vi "_PC_Pub ctrlRegistry.vi"(5 "type":enum16{"None", "Write", "Read"}(ring)=enum."Read", 7 "function":T1=enum."ExeStatu", 8 "error in (no error)":errorcluster, 10 "node":string, 11 "write value":variant) -> (0 "error out":errorcluster, 1 "Boolean output":bool, 2 "SZ output":string, 3 "DWORD outpur":u32)   [LabVIEW 2018]
uses:
  Ctl/RegistyFunc.ctl
  <vilib>/registry/registry.llb/Registry RtKey.ctl
  <vilib>/registry/registry.llb/Read Registry Value Simple U32.vi
  <vilib>/registry/registry.llb/Write Registry Value Simple U32.vi
  <vilib>/registry/registry.llb/Read Registry Value Simple STR.vi
  <vilib>/registry/registry.llb/Write Registry Value Simple STR.vi
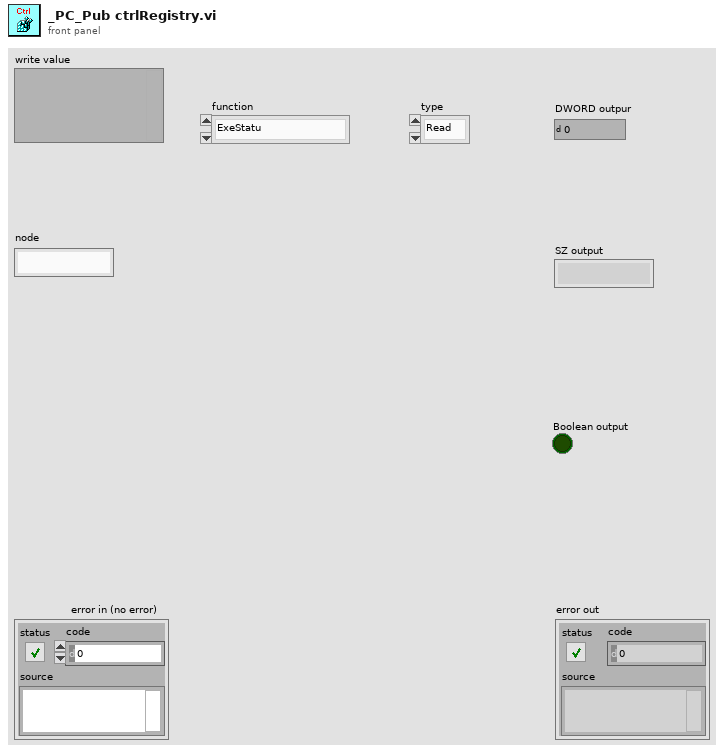
[diagram p1: front panel]
types:
  T1 = typedef "RegistyFunc.ctl" = enum16{"None", "FileAutoSave", "FileNoise", "FileSN", "ExeStatu", "WorkFolderPath", "MethodPath", "AVGItem", "LoopItem", "AutoRun", "BGColor", "LineColor", "LineWidth", "XGrid", "YGrid", "DeviceRefnum"}
  T2 = typedef "Registry RtKey.ctl" = enum32{"HKEY_CLASSES_ROOT", "HKEY_CURRENT_USER", "HKEY_LOCAL_MACHINE", "HKEY_USERS", "HKEY_PERFORMANCE_DATA", "HKEY_CURRENT_CONFIG", "HKEY_DYN_DATA"}
  T3 = typedef "Registry refnum.ctl" = refnum<k1>
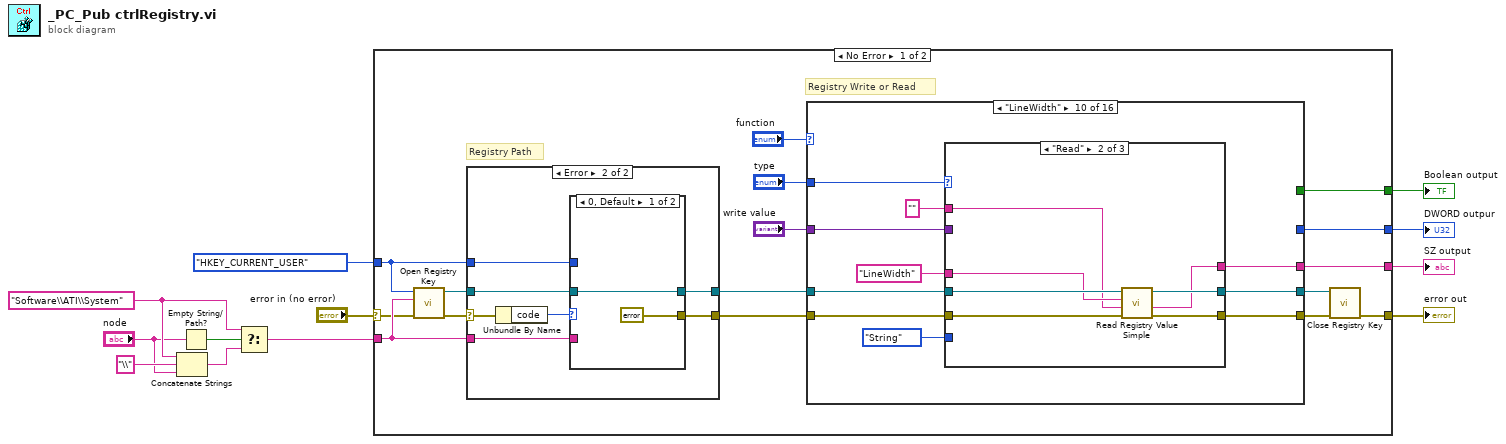
[diagram p0: block diagram]
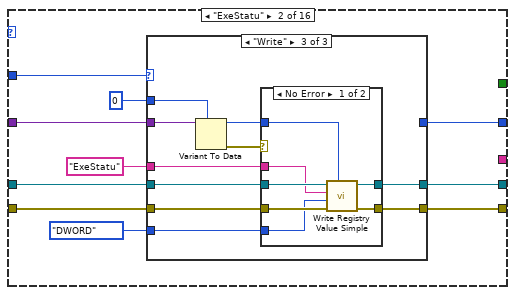
[diagram p3: hidden frame]
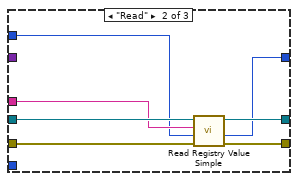
[diagram p5: hidden frame]
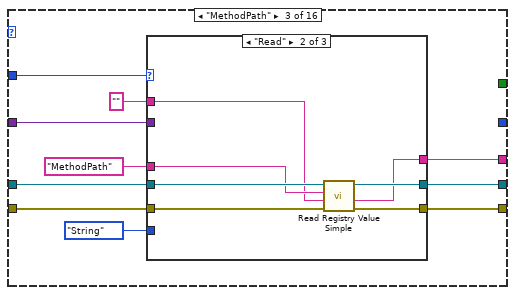
[diagram p7: hidden frame]
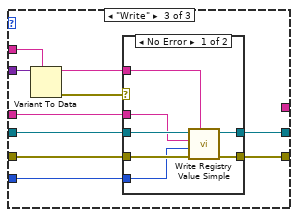
[diagram p9: hidden frame]
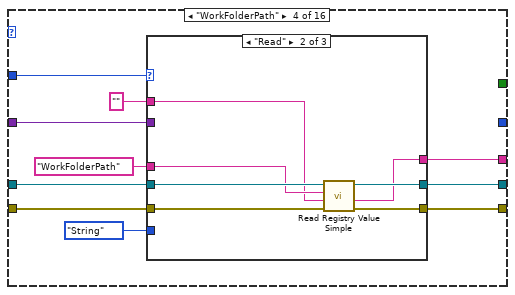
[diagram p11: hidden frame]
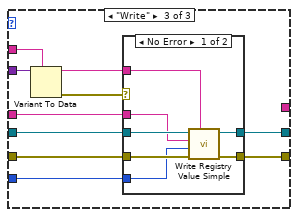
[diagram p13: hidden frame]
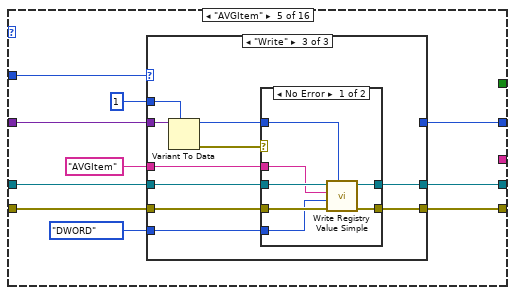
[diagram p15: hidden frame]
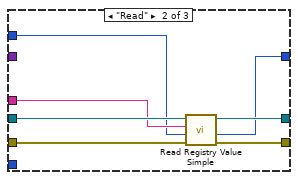
[diagram p17: hidden frame]
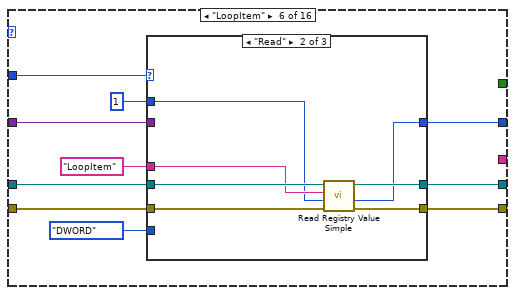
[diagram p19: hidden frame]
diagram:
  w9 = "Software\\ATI\\System" ("subkey")
  n1 = Concatenate Strings(w9, "\\" ("string"), "node") -> (w6:string)
  n2 = Empty String/Path?(string/path="node") -> (empty?=w10:bool)
  n3 = Select(t=w9, s=w10, f=w6) -> (s? t:f=w5:string)
  n4 = case shown="No Error" "error in (no error)" {
    selector: "error in (no error)" -> [w13 w636]
    tunnel: Registry_RtKey."HKEY_CURRENT_USER" ("root key (HKEY_LOCAL_MACHINE)") -> [w26 _]
    tunnel: [w18 w636] -> w11
    tunnel: w5 -> [w17 _]
    tunnel: [w16 _] -> w4
    tunnel: [w15 _] -> w3
    tunnel: [w14 _] -> w2
    frame No Error {
      # "Registry Path"
      # "Registry Write or Read"
      n5 = call <vilib>:"Open Registry Key.vi"("error in (no error)"=w13, "subkey"=w17, "root key (HKEY_LOCAL_MACHINE)"=w26) -> ("error out"=w28:errorcluster, "refnum out"=w27:T3)  [unwired: 7 in]
      n6 = case shown="Error" w28 {
        selector: w28 -> [w621 w629]
        tunnel: w27 -> [w622 w627]
        tunnel: w26 -> [_ w626]
        tunnel: w17 -> [_ w625]
        tunnel: [w622 w624] -> w22
        tunnel: [w621 w623] -> w21
        frame No Error {
        }
        frame Error {
          n7 = Unbundle By Name(w629) -> ("code"=w628:i32)
          n8 = case shown="0, Default" w628 {
            tunnel: w627 -> [w631 _]
            tunnel: w626 -> [_ w635]
            tunnel: w625 -> [_ w634]
            tunnel: [w631 w633] -> w624
            tunnel: [errorcluster {"status"=TRUE, "code"=5003, "source"=""} ("error out") w632] -> w623
            frame 0, Default {
            }
            frame -603 {
              n9 = call <vilib>:"Create Registry Key.vi"("subkey"=w634, "root key (HKEY_LOCAL_MACHINE)"=w635) -> ("error out"=w632:errorcluster, "refnum out"=w633:T3)  [unwired: 7 in, 1 out]
            }
          }
        }
      }
      n10 = case shown="\"LineWidth\"" "function" {
        tunnel: w22 -> [w30 w40 w78 w116 w154 w192 w230 w273 w311 w349 w387 w430 w473 w516 w554 w592]
        tunnel: [w30 w39 w77 w115 w153 w191 w229 w272 w310 w348 w386 w429 w472 w515 w553 w591] -> w24
        tunnel: [w29 w38 w76 w114 w152 w190 w228 w271 w309 w347 w385 w428 w471 w514 w552 w590] -> w23
        tunnel: w21 -> [w29 w35 w74 w112 w150 w188 w226 w269 w307 w345 w383 w426 w469 w512 w550 w588]
        tunnel: "type" -> [_ w37 w75 w113 w151 w189 w227 w270 w308 w346 w384 w427 w470 w513 w551 w589]
        tunnel: [_ w36 _ _ w145 w183 _ w264 _ _ _ _ _ _ _ _] -> w14
        tunnel: "write value" -> [_ w32 w71 w109 w147 w185 w223 w266 w304 w342 w380 w423 w466 w509 w547 w585]
        tunnel: [_ _ w69 w107 _ _ _ _ w302 w340 _ _ _ w507 w545 w583] -> w15
        tunnel: [_ _ _ _ _ _ w221 _ _ _ w378 w421 w464 _ _ _] -> w16
        frame "None", Default {
        }
        frame "ExeStatu" {
          n11 = case shown="\"Write\"" w37 {
            tunnel: w40 -> [w42 w49 w59]
            tunnel: [w42 w48 w57] -> w39
            tunnel: [w41 w47 w56] -> w38
            tunnel: w35 -> [w41 w46 w58]
            tunnel: "ExeStatu" ("value") -> [_ w45 w55]
            tunnel: [_ w44 _] -> w36
            tunnel: enum16{"String", "Binary", "DWORD"}."DWORD" ("simple data type") -> [_ _ w54]
            tunnel: w32 -> [_ _ w53]
            tunnel: u32 0 -> [_ w43 w50]
            frame "None", Default {
            }
            frame "Read" {
              n12 = call-poly <vilib>:"Read Registry Value Simple.vi"("error in (no error)"=w46, "default data"=w43, "value"=w45, "refnum"=w49) -> ("error out"=w47:errorcluster, "DWORD data"=w44:u32, "refnum out"=w48:T3)  [unwired: 2 in, 1 out]
            }
            frame "Write" {
              n13 = Variant To Data(type=w50, Variant=w53) -> (data=w52:u32, error out=w51:errorcluster)  [unwired: 1 in]
              n14 = case shown="No Error" w51 {
                tunnel: w59 -> [w66 w68]
                tunnel: w58 -> [w65 w67]
                tunnel: [w64 w68] -> w57
                tunnel: [w63 w67] -> w56
                tunnel: w55 -> [w62 _]
                tunnel: w54 -> [w61 _]
                tunnel: w52 -> [w60 _]
                frame No Error {
                  n15 = call-poly <vilib>:"Write Registry Value Simple.vi"("DWORD data"=w60, "error in (no error)"=w65, "simple data type"=w61, "value"=w62, "refnum"=w66) -> ("error out"=w63:errorcluster, "refnum out"=w64:T3)  [unwired: 3 in]
                }
                frame Error {
                }
              }
            }
          }
        }
        frame "MethodPath" {
          n16 = case shown="\"Read\"" w75 {
            tunnel: w78 -> [w80 w87 w97]
            tunnel: [w80 w86 w95] -> w77
            tunnel: [w79 w85 w94] -> w76
            tunnel: w74 -> [w79 w84 w96]
            tunnel: "MethodPath" ("value") -> [_ w83 w93]
            tunnel: enum16{"String", "Binary", "DWORD"}."String" ("simple data type") -> [_ _ w92]
            tunnel: w71 -> [_ _ w91]
            tunnel: "" -> [_ w82 w88]
            tunnel: [_ w81 _] -> w69
            frame "None", Default {
            }
            frame "Read" {
              n17 = call-poly <vilib>:"Read Registry Value Simple.vi"("error in (no error)"=w84, "default data"=w82, "value"=w83, "refnum"=w87) -> ("error out"=w85:errorcluster, "String/Binary data"=w81:string, "refnum out"=w86:T3)  [unwired: 2 in, 1 out]
            }
            frame "Write" {
              n18 = Variant To Data(type=w88, Variant=w91) -> (data=w90:string, error out=w89:errorcluster)  [unwired: 1 in]
              n19 = case shown="No Error" w89 {
                tunnel: w97 -> [w104 w106]
                tunnel: w96 -> [w103 w105]
                tunnel: [w102 w106] -> w95
                tunnel: [w101 w105] -> w94
                tunnel: w93 -> [w100 _]
                tunnel: w92 -> [w99 _]
                tunnel: w90 -> [w98 _]
                frame No Error {
                  n20 = call-poly <vilib>:"Write Registry Value Simple.vi"("String/Binary data"=w98, "error in (no error)"=w103, "simple data type"=w99, "value"=w100, "refnum"=w104) -> ("error out"=w101:errorcluster, "refnum out"=w102:T3)  [unwired: 3 in]
                }
                frame Error {
                }
              }
            }
          }
        }
        frame "WorkFolderPath" {
          n21 = case shown="\"Read\"" w113 {
            tunnel: w116 -> [w118 w125 w135]
            tunnel: [w118 w124 w133] -> w115
            tunnel: [w117 w123 w132] -> w114
            tunnel: w112 -> [w117 w122 w134]
            tunnel: "WorkFolderPath" ("value") -> [_ w121 w131]
            tunnel: enum16{"String", "Binary", "DWORD"}."String" ("simple data type") -> [_ _ w130]
            tunnel: w109 -> [_ _ w129]
            tunnel: "" -> [_ w120 w126]
            tunnel: [_ w119 _] -> w107
            frame "None", Default {
            }
            frame "Read" {
              n22 = call-poly <vilib>:"Read Registry Value Simple.vi"("error in (no error)"=w122, "default data"=w120, "value"=w121, "refnum"=w125) -> ("error out"=w123:errorcluster, "String/Binary data"=w119:string, "refnum out"=w124:T3)  [unwired: 2 in, 1 out]
            }
            frame "Write" {
              n23 = Variant To Data(type=w126, Variant=w129) -> (data=w128:string, error out=w127:errorcluster)  [unwired: 1 in]
              n24 = case shown="No Error" w127 {
                tunnel: w135 -> [w142 w144]
                tunnel: w134 -> [w141 w143]
                tunnel: [w140 w144] -> w133
                tunnel: [w139 w143] -> w132
                tunnel: w131 -> [w138 _]
                tunnel: w130 -> [w137 _]
                tunnel: w128 -> [w136 _]
                frame No Error {
                  n25 = call-poly <vilib>:"Write Registry Value Simple.vi"("String/Binary data"=w136, "error in (no error)"=w141, "simple data type"=w137, "value"=w138, "refnum"=w142) -> ("error out"=w139:errorcluster, "refnum out"=w140:T3)  [unwired: 3 in]
                }
                frame Error {
                }
              }
            }
          }
        }
        frame "AVGItem" {
          n26 = case shown="\"Write\"" w151 {
            tunnel: w154 -> [w156 w163 w173]
            tunnel: [w156 w162 w171] -> w153
            tunnel: [w155 w161 w170] -> w152
            tunnel: w150 -> [w155 w160 w172]
            tunnel: "AVGItem" ("value") -> [_ w159 w169]
            tunnel: enum16{"String", "Binary", "DWORD"}."DWORD" ("simple data type") -> [_ _ w168]
            tunnel: w147 -> [_ _ w167]
            tunnel: u32 1 -> [_ w158 w164]
            tunnel: [_ w157 _] -> w145
            frame "None", Default {
            }
            frame "Read" {
              n27 = call-poly <vilib>:"Read Registry Value Simple.vi"("error in (no error)"=w160, "default data"=w158, "value"=w159, "refnum"=w163) -> ("error out"=w161:errorcluster, "DWORD data"=w157:u32, "refnum out"=w162:T3)  [unwired: 2 in, 1 out]
            }
            frame "Write" {
              n28 = Variant To Data(type=w164, Variant=w167) -> (data=w166:u32, error out=w165:errorcluster)  [unwired: 1 in]
              n29 = case shown="No Error" w165 {
                tunnel: w173 -> [w180 w182]
                tunnel: w172 -> [w179 w181]
                tunnel: [w178 w182] -> w171
                tunnel: [w177 w181] -> w170
                tunnel: w169 -> [w176 _]
                tunnel: w168 -> [w175 _]
                tunnel: w166 -> [w174 _]
                frame No Error {
                  n30 = call-poly <vilib>:"Write Registry Value Simple.vi"("DWORD data"=w174, "error in (no error)"=w179, "simple data type"=w175, "value"=w176, "refnum"=w180) -> ("error out"=w177:errorcluster, "refnum out"=w178:T3)  [unwired: 3 in]
                }
                frame Error {
                }
              }
            }
          }
        }
        frame "LoopItem" {
          n31 = case shown="\"Read\"" w189 {
            tunnel: w192 -> [w194 w201 w211]
            tunnel: [w194 w200 w209] -> w191
            tunnel: [w193 w199 w208] -> w190
            tunnel: w188 -> [w193 w198 w210]
            tunnel: "LoopItem" ("value") -> [_ w197 w207]
            tunnel: enum16{"String", "Binary", "DWORD"}."DWORD" ("simple data type") -> [_ _ w206]
            tunnel: w185 -> [_ _ w205]
            tunnel: u32 1 -> [_ w196 w202]
            tunnel: [_ w195 _] -> w183
            frame "None", Default {
            }
            frame "Read" {
              n32 = call-poly <vilib>:"Read Registry Value Simple.vi"("error in (no error)"=w198, "default data"=w196, "value"=w197, "refnum"=w201) -> ("error out"=w199:errorcluster, "DWORD data"=w195:u32, "refnum out"=w200:T3)  [unwired: 2 in, 1 out]
            }
            frame "Write" {
              n33 = Variant To Data(type=w202, Variant=w205) -> (data=w204:u32, error out=w203:errorcluster)  [unwired: 1 in]
              n34 = case shown="No Error" w203 {
                tunnel: w211 -> [w218 w220]
                tunnel: w210 -> [w217 w219]
                tunnel: [w216 w220] -> w209
                tunnel: [w215 w219] -> w208
                tunnel: w207 -> [w214 _]
                tunnel: w206 -> [w213 _]
                tunnel: w204 -> [w212 _]
                frame No Error {
                  n35 = call-poly <vilib>:"Write Registry Value Simple.vi"("DWORD data"=w212, "error in (no error)"=w217, "simple data type"=w213, "value"=w214, "refnum"=w218) -> ("error out"=w215:errorcluster, "refnum out"=w216:T3)  [unwired: 3 in]
                }
                frame Error {
                }
              }
            }
          }
        }
        frame "AutoRun" {
          n36 = case shown="\"Read\"" w227 {
            tunnel: w230 -> [w232 w241 w251]
            tunnel: [w232 w240 w249] -> w229
            tunnel: [w231 w239 w248] -> w228
            tunnel: w226 -> [w231 w238 w250]
            tunnel: "AutoRun" ("value") -> [_ w237 w247]
            tunnel: enum16{"String", "Binary", "DWORD"}."String" ("simple data type") -> [_ _ w246]
            tunnel: w223 -> [_ _ w245]
            tunnel: FALSE -> [_ _ w242]
            tunnel: [_ w233 _] -> w221
            frame "None", Default {
            }
            frame "Read" {
              n37 = call-poly <vilib>:"Read Registry Value Simple.vi"("error in (no error)"=w238, "default data"="" ("value"), "value"=w237, "refnum"=w241) -> ("error out"=w239:errorcluster, "String/Binary data"=w235:string, "refnum out"=w240:T3)  [unwired: 2 in, 1 out]
              n38 = Equal?(x="T", y=w235) -> (x = y?=w233:bool)
            }
            frame "Write" {
              n39 = Variant To Data(type=w242, Variant=w245) -> (data=w244:bool, error out=w243:errorcluster)  [unwired: 1 in]
              n40 = case shown="No Error" w243 {
                tunnel: w251 -> [w261 w263]
                tunnel: w250 -> [w260 w262]
                tunnel: [w259 w263] -> w249
                tunnel: [w258 w262] -> w248
                tunnel: w247 -> [w257 _]
                tunnel: w246 -> [w256 _]
                tunnel: w244 -> [w255 _]
                frame No Error {
                  n41 = Select(t="T", s=w255, f="F") -> (s? t:f=w252:string)
                  n42 = call-poly <vilib>:"Write Registry Value Simple.vi"("String/Binary data"=w252, "error in (no error)"=w260, "simple data type"=w256, "value"=w257, "refnum"=w261) -> ("error out"=w258:errorcluster, "refnum out"=w259:T3)  [unwired: 3 in]
                }
                frame Error {
                }
              }
            }
          }
        }
        frame "BGColor" {
          n43 = case shown="\"Read\"" w270 {
            tunnel: w273 -> [w275 w282 w292]
            tunnel: [w275 w281 w290] -> w272
            tunnel: [w274 w280 w289] -> w271
            tunnel: w269 -> [w274 w279 w291]
            tunnel: "BGColor" ("value") -> [_ w278 w288]
            tunnel: enum16{"String", "Binary", "DWORD"}."DWORD" ("simple data type") -> [_ _ w287]
            tunnel: w266 -> [_ _ w286]
            tunnel: u32 0 -> [_ w277 w283]
            tunnel: [_ w276 _] -> w264
            frame "None", Default {
            }
            frame "Read" {
              n44 = call-poly <vilib>:"Read Registry Value Simple.vi"("error in (no error)"=w279, "default data"=w277, "value"=w278, "refnum"=w282) -> ("error out"=w280:errorcluster, "DWORD data"=w276:u32, "refnum out"=w281:T3)  [unwired: 2 in, 1 out]
            }
            frame "Write" {
              n45 = Variant To Data(type=w283, Variant=w286) -> (data=w285:u32, error out=w284:errorcluster)  [unwired: 1 in]
              n46 = case shown="No Error" w284 {
                tunnel: w292 -> [w299 w301]
                tunnel: w291 -> [w298 w300]
                tunnel: [w297 w301] -> w290
                tunnel: [w296 w300] -> w289
                tunnel: w288 -> [w295 _]
                tunnel: w287 -> [w294 _]
                tunnel: w285 -> [w293 _]
                frame No Error {
                  n47 = call-poly <vilib>:"Write Registry Value Simple.vi"("DWORD data"=w293, "error in (no error)"=w298, "simple data type"=w294, "value"=w295, "refnum"=w299) -> ("error out"=w296:errorcluster, "refnum out"=w297:T3)  [unwired: 3 in]
                }
                frame Error {
                }
              }
            }
          }
        }
        frame "LineColor" {
          n48 = case shown="\"Write\"" w308 {
            tunnel: w311 -> [w313 w320 w330]
            tunnel: [w313 w319 w328] -> w310
            tunnel: [w312 w318 w327] -> w309
            tunnel: w307 -> [w312 w317 w329]
            tunnel: "LineColor" ("value") -> [_ w316 w326]
            tunnel: enum16{"String", "Binary", "DWORD"}."String" ("simple data type") -> [_ _ w325]
            tunnel: w304 -> [_ _ w324]
            tunnel: "" -> [_ w315 w321]
            tunnel: [_ w314 _] -> w302
            frame "None", Default {
            }
            frame "Read" {
              n49 = call-poly <vilib>:"Read Registry Value Simple.vi"("error in (no error)"=w317, "default data"=w315, "value"=w316, "refnum"=w320) -> ("error out"=w318:errorcluster, "String/Binary data"=w314:string, "refnum out"=w319:T3)  [unwired: 2 in, 1 out]
            }
            frame "Write" {
              n50 = Variant To Data(type=w321, Variant=w324) -> (data=w323:string, error out=w322:errorcluster)  [unwired: 1 in]
              n51 = case shown="Error" w322 {
                tunnel: w330 -> [w337 w339]
                tunnel: w329 -> [w336 w338]
                tunnel: [w335 w339] -> w328
                tunnel: [w334 w338] -> w327
                tunnel: w326 -> [w333 _]
                tunnel: w325 -> [w332 _]
                tunnel: w323 -> [w331 _]
                frame No Error {
                  n52 = call-poly <vilib>:"Write Registry Value Simple.vi"("String/Binary data"=w331, "error in (no error)"=w336, "simple data type"=w332, "value"=w333, "refnum"=w337) -> ("error out"=w334:errorcluster, "refnum out"=w335:T3)  [unwired: 3 in]
                }
                frame Error {
                }
              }
            }
          }
        }
        frame "LineWidth" {
          n53 = case shown="\"Read\"" w346 {
            tunnel: w349 -> [w351 w358 w368]
            tunnel: [w351 w357 w366] -> w348
            tunnel: [w350 w356 w365] -> w347
            tunnel: w345 -> [w350 w355 w367]
            tunnel: "LineWidth" ("value") -> [_ w354 w364]
            tunnel: enum16{"String", "Binary", "DWORD"}."String" ("simple data type") -> [_ _ w363]
            tunnel: w342 -> [_ _ w362]
            tunnel: "" -> [_ w353 w359]
            tunnel: [_ w352 _] -> w340
            frame "None", Default {
            }
            frame "Read" {
              n54 = call-poly <vilib>:"Read Registry Value Simple.vi"("error in (no error)"=w355, "default data"=w353, "value"=w354, "refnum"=w358) -> ("error out"=w356:errorcluster, "String/Binary data"=w352:string, "refnum out"=w357:T3)  [unwired: 2 in, 1 out]
            }
            frame "Write" {
              n55 = Variant To Data(type=w359, Variant=w362) -> (data=w361:string, error out=w360:errorcluster)  [unwired: 1 in]
              n56 = case shown="No Error" w360 {
                tunnel: w368 -> [w375 w377]
                tunnel: w367 -> [w374 w376]
                tunnel: [w373 w377] -> w366
                tunnel: [w372 w376] -> w365
                tunnel: w364 -> [w371 _]
                tunnel: w363 -> [w370 _]
                tunnel: w361 -> [w369 _]
                frame No Error {
                  n57 = call-poly <vilib>:"Write Registry Value Simple.vi"("String/Binary data"=w369, "error in (no error)"=w374, "simple data type"=w370, "value"=w371, "refnum"=w375) -> ("error out"=w372:errorcluster, "refnum out"=w373:T3)  [unwired: 3 in]
                }
                frame Error {
                }
              }
            }
          }
        }
        frame "XGrid" {
          n58 = case shown="\"Read\"" w384 {
            tunnel: w387 -> [w389 w398 w408]
            tunnel: [w389 w397 w406] -> w386
            tunnel: [w388 w396 w405] -> w385
            tunnel: w383 -> [w388 w395 w407]
            tunnel: "XGrid" ("value") -> [_ w394 w404]
            tunnel: enum16{"String", "Binary", "DWORD"}."String" ("simple data type") -> [_ _ w403]
            tunnel: w380 -> [_ _ w402]
            tunnel: FALSE -> [_ _ w399]
            tunnel: [_ w390 _] -> w378
            frame "None", Default {
            }
            frame "Read" {
              n59 = call-poly <vilib>:"Read Registry Value Simple.vi"("error in (no error)"=w395, "default data"="" ("value"), "value"=w394, "refnum"=w398) -> ("error out"=w396:errorcluster, "String/Binary data"=w392:string, "refnum out"=w397:T3)  [unwired: 2 in, 1 out]
              n60 = Equal?(x="T", y=w392) -> (x = y?=w390:bool)
            }
            frame "Write" {
              n61 = Variant To Data(type=w399, Variant=w402) -> (data=w401:bool, error out=w400:errorcluster)  [unwired: 1 in]
              n62 = case shown="No Error" w400 {
                tunnel: w408 -> [w418 w420]
                tunnel: w407 -> [w417 w419]
                tunnel: [w416 w420] -> w406
                tunnel: [w415 w419] -> w405
                tunnel: w404 -> [w414 _]
                tunnel: w403 -> [w413 _]
                tunnel: w401 -> [w412 _]
                frame No Error {
                  n63 = Select(t="T", s=w412, f="F") -> (s? t:f=w409:string)
                  n64 = call-poly <vilib>:"Write Registry Value Simple.vi"("String/Binary data"=w409, "error in (no error)"=w417, "simple data type"=w413, "value"=w414, "refnum"=w418) -> ("error out"=w415:errorcluster, "refnum out"=w416:T3)  [unwired: 3 in]
                }
                frame Error {
                }
              }
            }
          }
        }
        frame "YGrid" {
          n65 = case shown="\"Read\"" w427 {
            tunnel: w430 -> [w432 w441 w451]
            tunnel: [w432 w440 w449] -> w429
            tunnel: [w431 w439 w448] -> w428
            tunnel: w426 -> [w431 w438 w450]
            tunnel: "YGrid" ("value") -> [_ w437 w447]
            tunnel: enum16{"String", "Binary", "DWORD"}."String" ("simple data type") -> [_ _ w446]
            tunnel: w423 -> [_ _ w445]
            tunnel: FALSE -> [_ _ w442]
            tunnel: [_ w433 _] -> w421
            frame "None", Default {
            }
            frame "Read" {
              n66 = call-poly <vilib>:"Read Registry Value Simple.vi"("error in (no error)"=w438, "default data"="" ("value"), "value"=w437, "refnum"=w441) -> ("error out"=w439:errorcluster, "String/Binary data"=w435:string, "refnum out"=w440:T3)  [unwired: 2 in, 1 out]
              n67 = Equal?(x="T", y=w435) -> (x = y?=w433:bool)
            }
            frame "Write" {
              n68 = Variant To Data(type=w442, Variant=w445) -> (data=w444:bool, error out=w443:errorcluster)  [unwired: 1 in]
              n69 = case shown="No Error" w443 {
                tunnel: w451 -> [w461 w463]
                tunnel: w450 -> [w460 w462]
                tunnel: [w459 w463] -> w449
                tunnel: [w458 w462] -> w448
                tunnel: w447 -> [w457 _]
                tunnel: w446 -> [w456 _]
                tunnel: w444 -> [w455 _]
                frame No Error {
                  n70 = Select(t="T", s=w455, f="F") -> (s? t:f=w452:string)
                  n71 = call-poly <vilib>:"Write Registry Value Simple.vi"("String/Binary data"=w452, "error in (no error)"=w460, "simple data type"=w456, "value"=w457, "refnum"=w461) -> ("error out"=w458:errorcluster, "refnum out"=w459:T3)  [unwired: 3 in]
                }
                frame Error {
                }
              }
            }
          }
        }
        frame "FileAutoSave" {
          n72 = case shown="\"Read\"" w470 {
            tunnel: w473 -> [w475 w484 w494]
            tunnel: [w475 w483 w492] -> w472
            tunnel: [w474 w482 w491] -> w471
            tunnel: w469 -> [w474 w481 w493]
            tunnel: "FileAutoSave" ("value") -> [_ w480 w490]
            tunnel: enum16{"String", "Binary", "DWORD"}."String" ("simple data type") -> [_ _ w489]
            tunnel: w466 -> [_ _ w488]
            tunnel: FALSE -> [_ _ w485]
            tunnel: [_ w476 _] -> w464
            frame "None", Default {
            }
            frame "Read" {
              n73 = call-poly <vilib>:"Read Registry Value Simple.vi"("error in (no error)"=w481, "default data"="" ("value"), "value"=w480, "refnum"=w484) -> ("error out"=w482:errorcluster, "String/Binary data"=w478:string, "refnum out"=w483:T3)  [unwired: 2 in, 1 out]
              n74 = Equal?(x="T", y=w478) -> (x = y?=w476:bool)
            }
            frame "Write" {
              n75 = Variant To Data(type=w485, Variant=w488) -> (data=w487:bool, error out=w486:errorcluster)  [unwired: 1 in]
              n76 = case shown="No Error" w486 {
                tunnel: w494 -> [w504 w506]
                tunnel: w493 -> [w503 w505]
                tunnel: [w502 w506] -> w492
                tunnel: [w501 w505] -> w491
                tunnel: w490 -> [w500 _]
                tunnel: w489 -> [w499 _]
                tunnel: w487 -> [w498 _]
                frame No Error {
                  n77 = Select(t="T", s=w498, f="F") -> (s? t:f=w495:string)
                  n78 = call-poly <vilib>:"Write Registry Value Simple.vi"("String/Binary data"=w495, "error in (no error)"=w503, "simple data type"=w499, "value"=w500, "refnum"=w504) -> ("error out"=w501:errorcluster, "refnum out"=w502:T3)  [unwired: 3 in]
                }
                frame Error {
                }
              }
            }
          }
        }
        frame "FileNoise" {
          n79 = case shown="\"Read\"" w513 {
            tunnel: w516 -> [w518 w525 w535]
            tunnel: [w518 w524 w533] -> w515
            tunnel: [w517 w523 w532] -> w514
            tunnel: w512 -> [w517 w522 w534]
            tunnel: "FileNoise" ("value") -> [_ w521 w531]
            tunnel: enum16{"String", "Binary", "DWORD"}."String" ("simple data type") -> [_ _ w530]
            tunnel: w509 -> [_ _ w529]
            tunnel: "" -> [_ w520 w526]
            tunnel: [_ w519 _] -> w507
            frame "None", Default {
            }
            frame "Read" {
              n80 = call-poly <vilib>:"Read Registry Value Simple.vi"("error in (no error)"=w522, "default data"=w520, "value"=w521, "refnum"=w525) -> ("error out"=w523:errorcluster, "String/Binary data"=w519:string, "refnum out"=w524:T3)  [unwired: 2 in, 1 out]
            }
            frame "Write" {
              n81 = Variant To Data(type=w526, Variant=w529) -> (data=w528:string, error out=w527:errorcluster)  [unwired: 1 in]
              n82 = case shown="No Error" w527 {
                tunnel: w535 -> [w542 w544]
                tunnel: w534 -> [w541 w543]
                tunnel: [w540 w544] -> w533
                tunnel: [w539 w543] -> w532
                tunnel: w531 -> [w538 _]
                tunnel: w530 -> [w537 _]
                tunnel: w528 -> [w536 _]
                frame No Error {
                  n83 = call-poly <vilib>:"Write Registry Value Simple.vi"("String/Binary data"=w536, "error in (no error)"=w541, "simple data type"=w537, "value"=w538, "refnum"=w542) -> ("error out"=w539:errorcluster, "refnum out"=w540:T3)  [unwired: 3 in]
                }
                frame Error {
                }
              }
            }
          }
        }
        frame "FileSN" {
          n84 = case shown="\"None\", Default" w551 {
            tunnel: w554 -> [w556 w563 w573]
            tunnel: [w556 w562 w571] -> w553
            tunnel: [w555 w561 w570] -> w552
            tunnel: w550 -> [w555 w560 w572]
            tunnel: "FileSN" ("value") -> [_ w559 w569]
            tunnel: enum16{"String", "Binary", "DWORD"}."String" ("simple data type") -> [_ _ w568]
            tunnel: w547 -> [_ _ w567]
            tunnel: "" -> [_ w558 w564]
            tunnel: [_ w557 _] -> w545
            frame "None", Default {
            }
            frame "Read" {
              n85 = call-poly <vilib>:"Read Registry Value Simple.vi"("error in (no error)"=w560, "default data"=w558, "value"=w559, "refnum"=w563) -> ("error out"=w561:errorcluster, "String/Binary data"=w557:string, "refnum out"=w562:T3)  [unwired: 2 in, 1 out]
            }
            frame "Write" {
              n86 = Variant To Data(type=w564, Variant=w567) -> (data=w566:string, error out=w565:errorcluster)  [unwired: 1 in]
              n87 = case shown="No Error" w565 {
                tunnel: w573 -> [w580 w582]
                tunnel: w572 -> [w579 w581]
                tunnel: [w578 w582] -> w571
                tunnel: [w577 w581] -> w570
                tunnel: w569 -> [w576 _]
                tunnel: w568 -> [w575 _]
                tunnel: w566 -> [w574 _]
                frame No Error {
                  n88 = call-poly <vilib>:"Write Registry Value Simple.vi"("String/Binary data"=w574, "error in (no error)"=w579, "simple data type"=w575, "value"=w576, "refnum"=w580) -> ("error out"=w577:errorcluster, "refnum out"=w578:T3)  [unwired: 3 in]
                }
                frame Error {
                }
              }
            }
          }
        }
        frame "DeviceRefnum" {
          n89 = case shown="\"Read\"" w589 {
            tunnel: w592 -> [w594 w601 w611]
            tunnel: [w594 w600 w609] -> w591
            tunnel: [w593 w599 w608] -> w590
            tunnel: w588 -> [w593 w598 w610]
            tunnel: "DeviceRefnum" ("value") -> [_ w597 w607]
            tunnel: enum16{"String", "Binary", "DWORD"}."String" ("simple data type") -> [_ _ w606]
            tunnel: w585 -> [_ _ w605]
            tunnel: "" -> [_ w596 w602]
            tunnel: [_ w595 _] -> w583
            frame "None", Default {
            }
            frame "Read" {
              n90 = call-poly <vilib>:"Read Registry Value Simple.vi"("error in (no error)"=w598, "default data"=w596, "value"=w597, "refnum"=w601) -> ("error out"=w599:errorcluster, "String/Binary data"=w595:string, "refnum out"=w600:T3)  [unwired: 2 in, 1 out]
            }
            frame "Write" {
              n91 = Variant To Data(type=w602, Variant=w605) -> (data=w604:string, error out=w603:errorcluster)  [unwired: 1 in]
              n92 = case shown="No Error" w603 {
                tunnel: w611 -> [w618 w620]
                tunnel: w610 -> [w617 w619]
                tunnel: [w616 w620] -> w609
                tunnel: [w615 w619] -> w608
                tunnel: w607 -> [w614 _]
                tunnel: w606 -> [w613 _]
                tunnel: w604 -> [w612 _]
                frame No Error {
                  n93 = call-poly <vilib>:"Write Registry Value Simple.vi"("String/Binary data"=w612, "error in (no error)"=w617, "simple data type"=w613, "value"=w614, "refnum"=w618) -> ("error out"=w615:errorcluster, "refnum out"=w616:T3)  [unwired: 3 in]
                }
                frame Error {
                }
              }
            }
          }
        }
      }
      n94 = call <vilib>:"Close Registry Key.vi"("error in (no error)"=w23, "refnum"=w24) -> ("error out"=w18:errorcluster)  [unwired: 5 in]
    }
    frame Error {
    }
  }
  "error out" <- w11
  "DWORD outpur" <- w2
  "SZ output" <- w3
  "Boolean output" <- w4
